vi "EminemExecuteLogic.vi"(8 "Ball Sensor B":bool, 9 "Ball Sensor A":bool, 10 "Shooter_B_Vel_RPM":dbl, 11 "Shooter_A_Vel_RPM":dbl) -> (0 "Box states":T1=enum."13-AmpDone", 1 "Shooter_Feed_Motor_Out":dbl, 2 "Shooter_B_Motor_Out":dbl, 3 "Shooter_A_Motor_Out":dbl)   [LabVIEW 2023]
uses:
  EminemStatesEnum.ctl
  <vilib>/Rock Robotics/WPI/ThirdParty/JAS_Junk/TrajLib/Trajectory_Library.lvlib
  <vilib>/Rock Robotics/WPI/ThirdParty/JAS_Junk/TrajLib/TypeDef/PID_ERROR_TOLERANCE.ctl
  EminemGlobals.vi
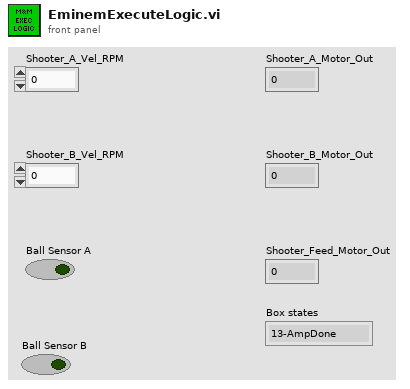
[diagram p1: front panel]
types:
  T1 = typedef "EminemStatesEnum.ctl" = enum16{"0-Init", "1-WaitForCmd", "2-Cancel", "3-ShootStart", "4-ShootRev", "5-ShootUpToSpd?", "6-ShootStartFeed&Timer", "7-ShootTimerOrSensorDone", "8-ShootDone", "9-AmpStart", "10-AmpUpToSpd?", "11-AmpStartFeed&Timer", "12-AmpTimerOrSensorDone", "13-AmpDone"}
  T2 = enum16{"Moving Average", "Low Pass 1st Order Butterworth", "Low Pass 2nd Order Butterworth", "High Pass 1st Order Butterworth", "High Pass 2nd Order Butterworth"}
  T3 = typedef "Trajectory_Library.lvlib/PID_ERROR_TOLERANCE.ctl" = cluster{"PositionTolerance":dbl, "VelocityTolerance":dbl}
  T4 = typedef "Trajectory_Library.lvlib/SIMPLE_MOTOR_FF.ctl" = cluster{"Ks":dbl, "Kv":dbl, "Ka":dbl, "KnInv":dbl}
  T5 = typedef "Trajectory_Library.lvlib/PID_ADV_LIMITS.ctl" = cluster{"MaxInput":dbl, "MinInput":dbl, "Continuous":bool, "MaxOutput":dbl, "MinOutput":dbl}
  T6 = typedef "Trajectory_Library.lvlib/PID_ADV_TUNING.ctl" = cluster{"Kf":dbl, "Kp":dbl, "Ki":dbl, "Kd":dbl, "MaximumIntegral":dbl, "MinimumIntegral":dbl, "Filter Derivative":bool, "IntegralZone":dbl}
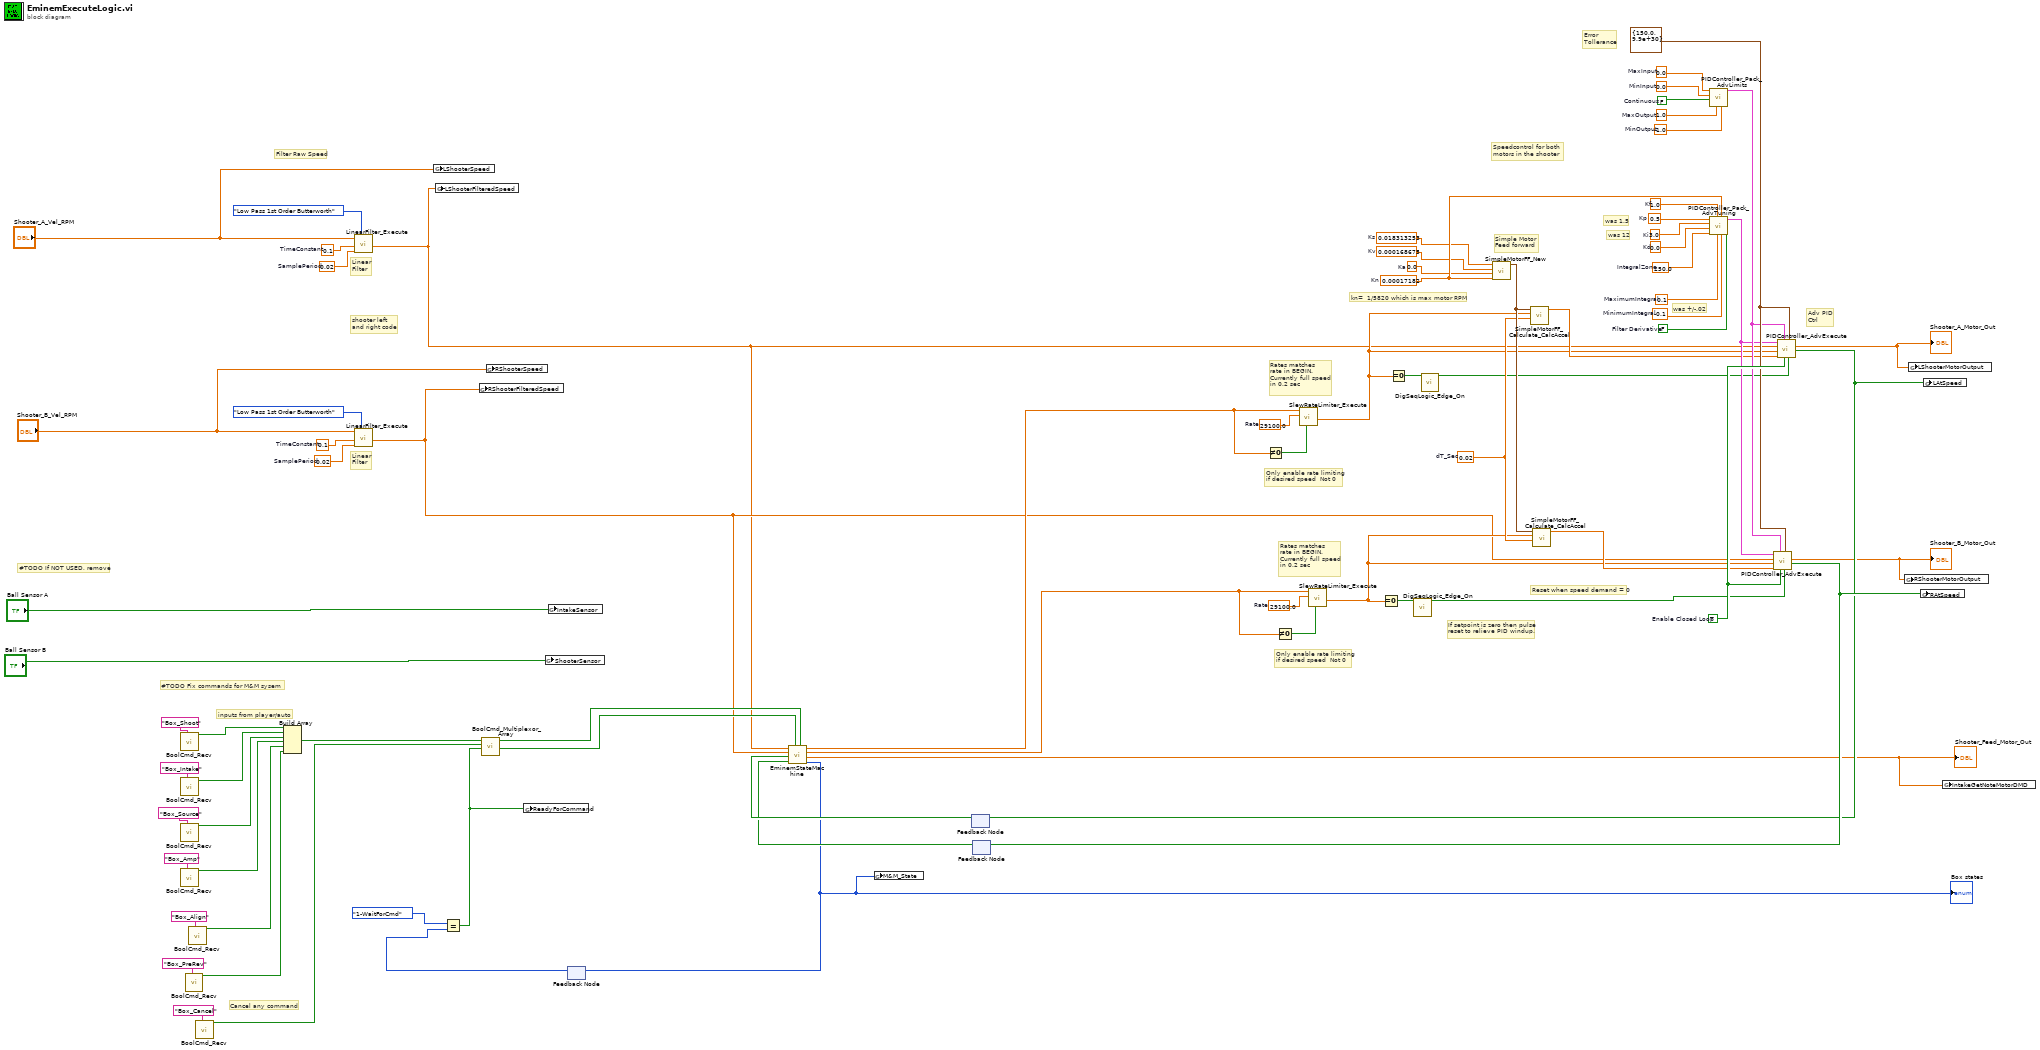
[diagram p0: block diagram]
diagram:
  w18 = 29100.0  # Rate
  w77 = 250.0  # IntegralZone
  w72 = 29100.0  # Rate
  w65 = 0.02  # SamplePeriod
  w66 = 0.1  # TimeConstant
  w62 = 0.02  # SamplePeriod
  w63 = 0.1  # TimeConstant
  w74 = TRUE  # Enable Closed Loop
  w60 = T3 {"PositionTolerance"=150.0, "VelocityTolerance"=9.9e+30} ("PID Error Tolerance")
  w48 = 0.00017182  # Kn
  w45 = 0.018313253  # Ks
  w46 = 0.000168675  # Kv
  w47 = 0.0  # Ka
  w50 = 0.5  # Kp
  w51 = 3.0  # Ki
  w52 = 0.0  # Kd
  w49 = 1.0  # Kf
  w53 = 0.1  # MaximumIntegral
  w54 = -0.1  # MinimumIntegral
  w55 = FALSE  # Filter Derivative
  w41 = 0.0  # MinInput
  w42 = FALSE  # Continuous
  w43 = 1.0  # MaxOutput
  w44 = -1.0  # MinOutput
  w40 = 0.0  # MaxInput
  w56 = 0.02  # dT_Sec
  # "Error \nTollerance"
  # "#TODO Fix commands for M&M sysem"
  # "#TODO If NOT USED, remove"
  # "Filter Raw Speed"
  # "Rates matches\nrate in BEGIN.  \nCurrently full speed\nin 0.2 sec"
  # "Only enable rate limiting\nif desired speed  Not 0"
  # "Reset when speed demand = 0"
  # "was 12"
  # "was 1.5"
  # "was +/-.02"
  # "If setpoint is zero then pulse\nreset to relieve PID windup."
  # "Rates matches\nrate in BEGIN.  \nCurrently full speed\nin 0.2 sec"
  # "Only enable rate limiting\nif desired speed  Not 0"
  # "inputs from player/auto"
  # "Linear\nFilter"
  # "Linear\nFilter"
  # "Speedcontrol for both \nmotors in the shooter"
  # "Simple Motor\nFeed forward"
  # "Adv PID\nCtrl"
  # "Cancel any command"
  # "kn=  1/5820 which is max motor RPM"
  # "shooter left \nand right code"
  n1 = call <vilib>:"BoolCmd_Recv.vi"("Command Name"="Box_Shoot") -> ("New Request"=w33:bool)  [unwired: 9 in, 1 out]
  n2 = call <vilib>:"BoolCmd_Recv.vi"("Command Name"="Box_Intake") -> ("New Request"=w32:bool)  [unwired: 9 in, 1 out]
  n3 = call <vilib>:"BoolCmd_Recv.vi"("Command Name"="Box_Source") -> ("New Request"=w29:bool)  [unwired: 9 in, 1 out]
  n4 = call <vilib>:"BoolCmd_Recv.vi"("Command Name"="Box_Amp") -> ("New Request"=w28:bool)  [unwired: 9 in, 1 out]
  n5 = call <vilib>:"BoolCmd_Recv.vi"("Command Name"="Box_PreRev") -> ("New Request"=w76:bool)  [unwired: 9 in, 1 out]
  n6 = call <vilib>:"BoolCmd_Recv.vi"("Command Name"="Box_Align") -> ("New Request"=w69:bool)  [unwired: 9 in, 1 out]
  n7 = call <vilib>:"BoolCmd_Recv.vi"("Command Name"="Box_Cancel") -> ("New Request"=w35:bool)  [unwired: 9 in, 1 out]
  n8 = Build Array(w33, w32, w29, w28, w69, w76) -> (w34:bool[])
  n9 = call <vilib>:"LinearFilter_Execute.vi"("Filter Type"=T2."Low Pass 1st Order Butterworth", "SamplePeriod"=w65, "TimeConstant"=w66, "Input"="Shooter_A_Vel_RPM") -> ("Output"=w1:dbl)  [unwired: 6 in, 1 out]
  n10 = call <vilib>:"LinearFilter_Execute.vi"("Filter Type"=T2."Low Pass 1st Order Butterworth", "SamplePeriod"=w62, "TimeConstant"=w63, "Input"="Shooter_B_Vel_RPM") -> ("Output"=w3:dbl)  [unwired: 6 in, 1 out]
  n11 = global write "EminemGlobals.vi" "LShooterSpeed"("Shooter_A_Vel_RPM") -> ()
  n12 = global write "EminemGlobals.vi" "LShooterFilteredSpeed"(w1) -> ()
  n13 = global write "EminemGlobals.vi" "RShooterFilteredSpeed"(w3) -> ()
  n14 = global write "EminemGlobals.vi" "RShooterSpeed"("Shooter_B_Vel_RPM") -> ()
  n15 = global write "EminemGlobals.vi" "ShooterSensor"("Ball Sensor B") -> ()
  n16 = global write "EminemGlobals.vi" "IntakeSensor"("Ball Sensor A") -> ()
  n17 = feedback #1() -> (w22:T1)  [unwired: 1 in]
  n18 = Equal?(x=EminemStatesEnum."1-WaitForCmd" ("Box states"), y=w22) -> (x = y?=w20:bool)
  n19 = call <vilib>:"BoolCmd_Multiplexor_Array.vi"("Ready"=w20, "Command Cancel"=w35, "Commands"=w34) -> ("Do Cancel"=w23:bool, "Do Command"=w24:bool[])  [unwired: 7 in]
  n20 = global write "EminemGlobals.vi" "ReadyForCommand"(w20) -> ()
  n21 = feedback #2() -> (w17:bool)  [unwired: 1 in]
  n22 = feedback #3() -> (w16:bool)  [unwired: 1 in]
  n23 = call "EminemStateMachine.vi"("EminemCommand"=w24, "EminemCancel"=w23, "LowerShoot_At_Speed"=w16, "UpperShoot_At_Speed"=w17, "LowerShoot_Speed_RPM"=w3, "UpperShoot_Speed_RPM"=w1) -> ("Box states"=w12:T1, "AmpAndFeed-MotorDmd"=w5:dbl, "LowerShooter-RPM_Dmd"=w15:dbl, "UpperShooterAndAmp-RPM_Dmd"=w14:dbl)  [unwired: 2 in]
  "Shooter_Feed_Motor_Out" <- w5
  "Box states" <- w12
  n24 = feedback-in #1(w12) -> ()
  n25 = global write "EminemGlobals.vi" "M&M_State"(w12) -> ()
  n26 = Not Equal To 0?(x=w14) -> (x != 0?=w19:bool)
  n27 = Not Equal To 0?(x=w15) -> (x != 0?=w73:bool)
  n28 = call <vilib>:"SlewRateLimiter_Execute.vi"("Enable"=w19, "PositiveRate"=w18, "Input"=w14) -> ("Output"=w13:dbl)  [unwired: 7 in, 1 out]
  n29 = call <vilib>:"SlewRateLimiter_Execute.vi"("Enable"=w73, "PositiveRate"=w72, "Input"=w15) -> ("Output"=w25:dbl)  [unwired: 7 in, 1 out]
  n30 = Equal To 0?(x=w25) -> (x = 0?=w70:bool)
  n31 = Equal To 0?(x=w13) -> (x = 0?=w27:bool)
  n32 = call <vilib>:"DigSeqLogic_Edge_On.vi"("Input"=w70) -> ("On Edge"=w71:bool)  [unwired: 10 in]
  n33 = call <vilib>:"DigSeqLogic_Edge_On.vi"("Input"=w27) -> ("On Edge"=w26:bool)  [unwired: 10 in]
  n34 = call <vilib>:"SimpleMotorFF_New.vi"("Kn"=w48, "Ka"=w47, "Kv"=w46, "Ks"=w45) -> ("SIMPLE_MOTOR_FF"=w57:T4)  [unwired: 7 in]
  n35 = call <vilib>:"SimpleMotorFF_Calculate_CalcAccel.vi"("dT_Sec"=w56, "VelSp"=w13, "SIMPLE_MOTOR_FF"=w57) -> ("FeedForward"=w39:dbl)  [unwired: 8 in]
  n36 = call <vilib>:"SimpleMotorFF_Calculate_CalcAccel.vi"("dT_Sec"=w56, "VelSp"=w25, "SIMPLE_MOTOR_FF"=w57) -> ("FeedForward"=w61:dbl)  [unwired: 8 in]
  n37 = call <vilib>:"PIDController_Pack_AdvLimits.vi"("MinOutput"=w44, "MaxOutput"=w43, "Continuous"=w42, "MinInput"=w41, "MaxInput"=w40) -> ("Adv PID Limits"=w59:T5)  [unwired: 6 in]
  n38 = call <vilib>:"PIDController_Pack_AdvTuning.vi"("Filter Derivative"=w55, "MinimumIntegral"=w54, "Kn"=w48, "MaximumIntegral"=w53, "Kf"=w49, "IntegralZone"=w77, "Kd"=w52, "Ki"=w51, "Kp"=w50) -> ("Adv PID Tuning"=w58:T6)  [unwired: 2 in]
  n39 = call <vilib>:"PIDController_AdvExecute.vi"("Reset"=w71, "PID Error Tolerance"=w60, "Auto"=w74, "Adv PID Limits"=w59, "FF-FeedForward"=w61, "SP-SetPoint"=w25, "PV-Measurement"=w3, "Adv PID Tuning"=w58) -> ("AtSetpoint"=w11:bool, "CO-ControlOutput"=w6:dbl)  [unwired: 1 in, 1 out]
  "Shooter_B_Motor_Out" <- w6
  n40 = feedback-in #3(w11) -> ()
  n41 = call <vilib>:"PIDController_AdvExecute.vi"("Reset"=w26, "PID Error Tolerance"=w60, "Auto"=w74, "Adv PID Limits"=w59, "FF-FeedForward"=w39, "SP-SetPoint"=w13, "PV-Measurement"=w1, "Adv PID Tuning"=w58) -> ("AtSetpoint"=w10:bool, "CO-ControlOutput"=w7:dbl)  [unwired: 1 in, 1 out]
  "Shooter_A_Motor_Out" <- w7
  n42 = feedback-in #2(w10) -> ()
  n43 = global write "EminemGlobals.vi" "RShooterMotorOutput"(w6) -> ()
  n44 = global write "EminemGlobals.vi" "LShooterMotorOutput"(w7) -> ()
  n45 = global write "EminemGlobals.vi" "RAtSpeed"(w11) -> ()
  n46 = global write "EminemGlobals.vi" "LAtSpeed"(w10) -> ()
  n47 = global write "EminemGlobals.vi" "IntakeGetNoteMotorDMD"(w5) -> ()
